vi "Read_Write_INI.vi"(0 "Data_In":T1, 11 "Error_In":errorcluster, 13 "INI_Select":T3) -> (4 "Data_Out":T1, 15 "Error_Out":errorcluster)   [LabVIEW 2021]
doc: "Used to read and write the INI file."
uses:
  <vilib>/Utility/config.llb/NI_LVConfig.lvlib
  <vilib>/Utility/config.llb/Read Key (I32).vi
  <vilib>/Utility/config.llb/Write Key (I32).vi
  Controls/INI_Operation_Select.ctl
  Controls/Total_Cash_Count.ctl
  Controls/INI_Data.ctl
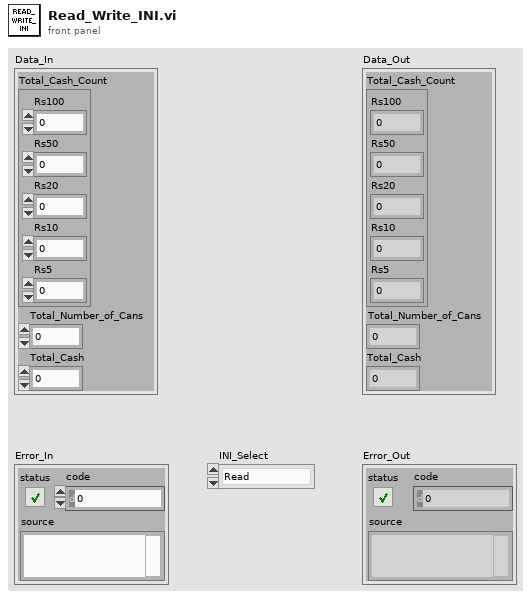
[diagram p1: front panel]
types:
  T1 = typedef "INI_Data.ctl" = cluster{"Total_Cash_Count":T2, "Total_Number_of_Cans":i32, "Total_Cash":i32}
  T2 = typedef "Total_Cash_Count.ctl" = cluster{"Rs100":i32, "Rs50":i32, "Rs20":i32, "Rs10":i32, "Rs5":i32}
  T3 = typedef "INI_Operation_Select.ctl" = enum16{"Read", "Write"}
  T4 = typedef "NI_LVConfig.lvlib/Config Data RefNum.ctl" = refnum<k1>
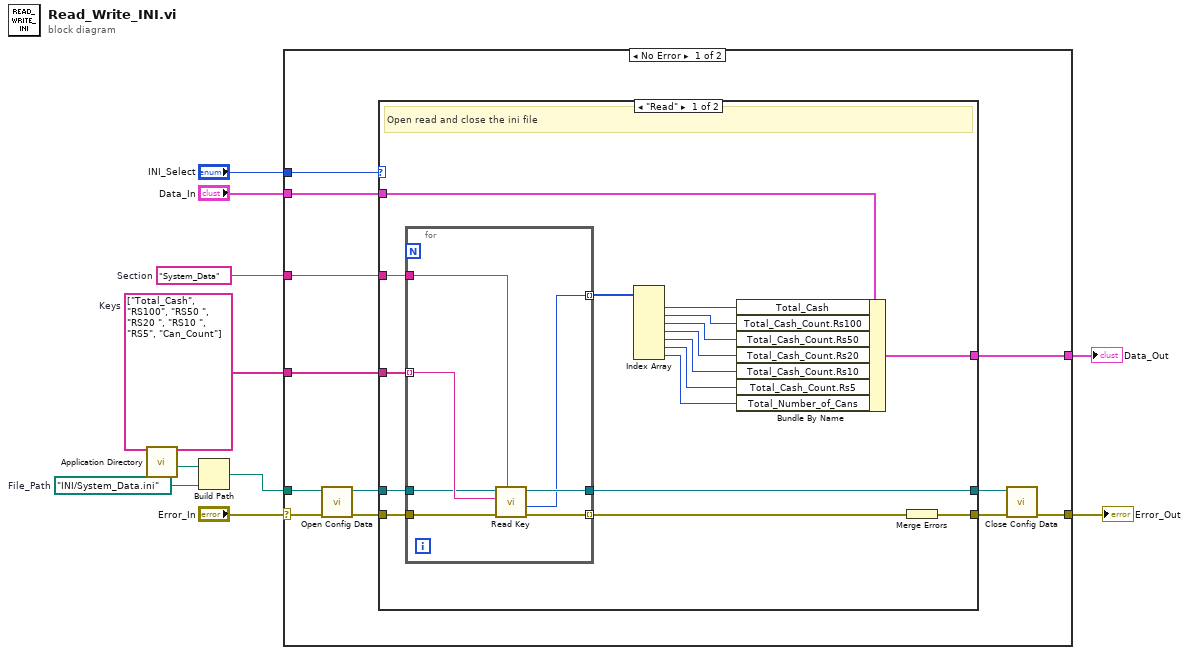
[diagram p0: block diagram]
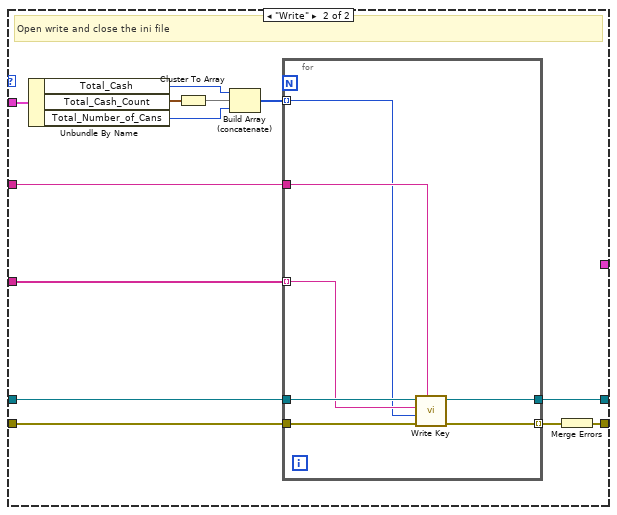
[diagram p2: hidden frame]
diagram:
  w2 = "System_Data"  # Section
  w3 = string[] ["Total_Cash", "RS100", "RS50 ", "RS20 ", "RS10 ", "RS5", "Can_Count"]  # Keys
  w5 = path "INI/System_Data.ini"  # File_Path
  n1 = call <vilib>:"Application Directory.vi"() -> ("Application Directory"=w6:path)
  n2 = Build Path(base path=w6, name or relative path=w5) -> (appended path=w4:path)
  n3 = case shown="No Error" "Error_In" {
    selector: "Error_In" -> [w18 w67]
    tunnel: [w22 w67] -> w10
    tunnel: w4 -> [w21 _]
    tunnel: "INI_Select" -> [w20 _]
    tunnel: "Data_In" -> [w13 _]
    tunnel: w3 -> [w19 _]
    tunnel: w2 -> [w12 _]
    tunnel: [w11 _] -> w1
    frame No Error {
      n4 = call <vilib>:"Open Config Data.vi"("error in (no error)"=w18, "configuration file path"=w21) -> ("error out"=w17:errorcluster, "refnum"=w16:T4)  [unwired: 7 in, 1 out]
      n5 = case shown="\"Read\"" w20 {
        tunnel: w17 -> [w38 w58]
        tunnel: [w34 w55] -> w15
        tunnel: w19 -> [w39 w54]
        tunnel: w16 -> [w37 w59]
        tunnel: [w36 w57] -> w14
        tunnel: w13 -> [w32 w48]
        tunnel: w12 -> [w33 w53]
        tunnel: [w23 _] -> w11
        frame "Read" {
          # "Open read and close the ini file"
          n6 = for {
            tunnel: w39 -> [w46] mode=indexing
            tunnel: w38 -> [w45]
            tunnel: [w42] -> w35 mode=indexing
            tunnel: w33 -> [w41]
            tunnel: [w40] -> w31 mode=indexing
            tunnel: w37 -> [w44]
            tunnel: [w43] -> w36
            n7 = call-poly <vilib>:"Read Key.vi"("section"=w41, "error in (no error)"=w45, "key"=w46, "refnum"=w44) -> ("error out"=w42:errorcluster, "value"=w40:i32, "refnum out"=w43:T4)  [unwired: 4 in, 1 out]
          }
          n8 = Index Array(array=w31) -> (element #1=w30:i32, element #2=w29:i32, element #3=w28:i32, element #4=w27:i32, element #5=w26:i32, element #6=w25:i32, element #7=w24:i32)  [unwired: 7 in]
          n9 = Bundle By Name(cluster=w32, "Total_Cash"=w30, "Total_Cash_Count.Rs100"=w29, "Total_Cash_Count.Rs50"=w28, "Total_Cash_Count.Rs20"=w27, "Total_Cash_Count.Rs10"=w26, "Total_Cash_Count.Rs5"=w25, "Total_Number_of_Cans"=w24) -> (w23:T1)
          n10 = Merge Errors(w35) -> (w34:errorcluster)
        }
        frame "Write" {
          # "Open write and close the ini file"
          n11 = Unbundle By Name(w48) -> ("Total_Cash"=w49:i32, "Total_Cash_Count"=w51:T2, "Total_Number_of_Cans"=w52:i32)
          n12 = Cluster To Array(cluster=w51) -> (array=w50:i32[])
          n13 = Build Array (concatenate)(w49, w50, w52) -> (w47:i32[])
          n14 = for {
            tunnel: w58 -> [w65]
            tunnel: [w63] -> w56 mode=indexing
            tunnel: w54 -> [w62] mode=indexing
            tunnel: w53 -> [w61]
            tunnel: w47 -> [w60] mode=indexing
            tunnel: w59 -> [w66]
            tunnel: [w64] -> w57
            n15 = call-poly <vilib>:"Write Key.vi"("section"=w61, "error in (no error)"=w65, "value"=w60, "key"=w62, "refnum"=w66) -> ("error out"=w63:errorcluster, "refnum out"=w64:T4)  [unwired: 4 in, 1 out]
          }
          n16 = Merge Errors(w56) -> (w55:errorcluster)
        }
      }
      n17 = call <vilib>:"Close Config Data.vi"("error in (no error)"=w15, "refnum"=w14) -> ("error out"=w22:errorcluster)  [unwired: 8 in, 1 out]
    }
    frame Error {
    }
  }
  "Error_Out" <- w10
  "Data_Out" <- w1
